vi "Obtain.vi"(8 "error in (no error)":errorcluster) -> (0 "error out":errorcluster, 3 "Get Controls out":refnum<class "Get Controls.lvclass">)   [LabVIEW 2020, in "Msg.lvlib" / "Get Controls.lvclass"]
doc: "Obtain a queue and populate the private data with the created queue."
uses:
  Get Controls.lvclass
  Controls/Ctl_Control Element.ctl
  Get Controls.lvclass/Get Controls.ctl
  Msg.lvlib
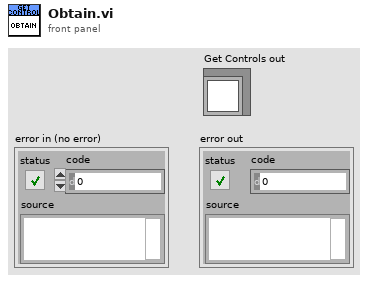
[diagram p1: front panel]
types:
  T1 = typedef "Msg.lvlib/Ctl_Control Element.ctl" = cluster{"Index":i32, "Label":string, "Value":variant}
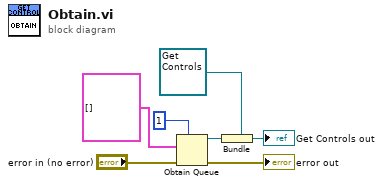
[diagram p0: block diagram]
diagram:
  n1 = Obtain Queue(max queue size (-1, unlimited)=1, element data type=T1[] [] ("Control Element Array"), error in (no error)="error in (no error)") -> (queue out=w2:refnum<queue>, error out=→"error out":errorcluster)  [unwired: 2 in, 1 out]
  n2 = Bundle(cluster=refnum<class "Get Controls.lvclass"> refnum ("Get Controls in"), w2) -> (→"Get Controls out":refnum<class "Get Controls.lvclass">)
